vi "Initialize Master.vi"(8 "error in":errorcluster, 11 "Serial Master in":refnum<class "Serial Master.lvclass">) -> (0 "error out":errorcluster, 3 "Serial Master out":refnum<class "Serial Master.lvclass">)   [LabVIEW 2021, in "Serial Master.lvclass"]
doc: "This provides an interface for the master to open a connection to the slave."
uses:
  Serial Master.lvclass
  Serial Master.lvclass/Serial Master.ctl
  Read timeout.vi
  Read data bits.vi
  Read VISA resource name.vi
  Read Baud Rate.vi
  Read Parity.vi
  Read Flow Control.vi
  Network Protocol.lvclass
  Transmission Data Unit/Transmission Data Unit.lvclass
  Network Interface/Network Interface.lvclass
  D:/my_projects/projects/Algorithms/Labview/21/Modbus_v121c/Network Protocol/Network Master/Network Master.lvclass
  D:/my_projects/projects/Algorithms/Labview/21/Modbus_v121c/Network Protocol/Network Protocol.lvclass
  D:/my_projects/projects/Algorithms/Labview/21/Modbus_v121c/Network Protocol/Network Master/Serial/Serial Master.lvclass
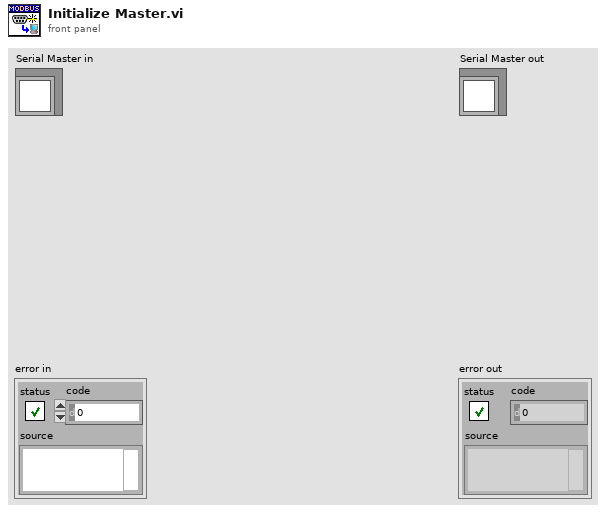
[diagram p1: front panel]
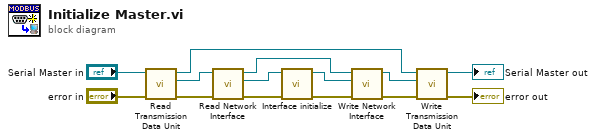
[diagram p0: block diagram]
diagram:
  n1 = call "Read Transmission Data Unit.vi"("error in (no error)"="error in", "Network Protocol in"="Serial Master in") -> ("error out"=w9:errorcluster, "Transmission Data Unit"=w14:refnum<class "Transmission Data Unit.lvclass">, "Network Protocol out"=w5:refnum<class "Serial Master.lvclass">)  [unwired: 7 in]
  n2 = call "Read Network Interface.vi"("error in (no error)"=w9, "Transmission Data Unit in"=w14) -> ("error out"=w8:errorcluster, "Network Interface"=w13:refnum<class "Network Interface.lvclass">, "Transmission Data Unit out"=w10:refnum<class "Transmission Data Unit.lvclass">)  [unwired: 7 in]
  n3 = call-dynamic "Interface initialize.vi"("error in"=w8, "interface in"=w13) -> ("error out"=w7:errorcluster, "interface out"=w12:refnum<class "Network Interface.lvclass">)  [unwired: 8 in]
  n4 = call "Write Network Interface.vi"("error in (no error)"=w7, "Network Interface"=w12, "Transmission Data Unit in"=w10) -> ("error out"=w6:errorcluster, "Transmission Data Unit out"=w11:refnum<class "Transmission Data Unit.lvclass">)  [unwired: 7 in]
  n5 = call "Write Transmission Data Unit.vi"("error in (no error)"=w6, "Transmission Data Unit"=w11, "Network Protocol in"=w5) -> ("error out"=→"error out":errorcluster, "Network Protocol out"=→"Serial Master out":refnum<class "Serial Master.lvclass">)  [unwired: 7 in]
